vi "Check Formulas Alias Name.vi"(6 "Reserved Keywords":string[](array[string])=["All_Photons", "F_D^D", "F_D^_A", "F_A^_D", "F_A^A", "F_D^M", "F_A^M", "Donor", "Acceptor", "FRET", "ALEX", "t_burst", "B_All", "B_D^D", "B_D^A", "B_A^D", "B_A^A", "B^D", "B^A"], 8 "Descriptions Array in":string[](array[string]), 9 "Definitions Array in":string[](array[string]), 10 "Aliases Array in":string[](array[string]), 11 "Alias Definition":T1) -> (0 "Descriptions Array out":string[](array[string]), 1 "Definitions Array out":string[](array[string]), 2 "Aliases Array out":string[](array[string]), 3 "Selected Alias":i32)   [LabVIEW 2021, in "Formula.lvlib"]
uses:
  Formula.lvlib
  Formula Alias Definition.ctl
  GUI/GUI.lvlib
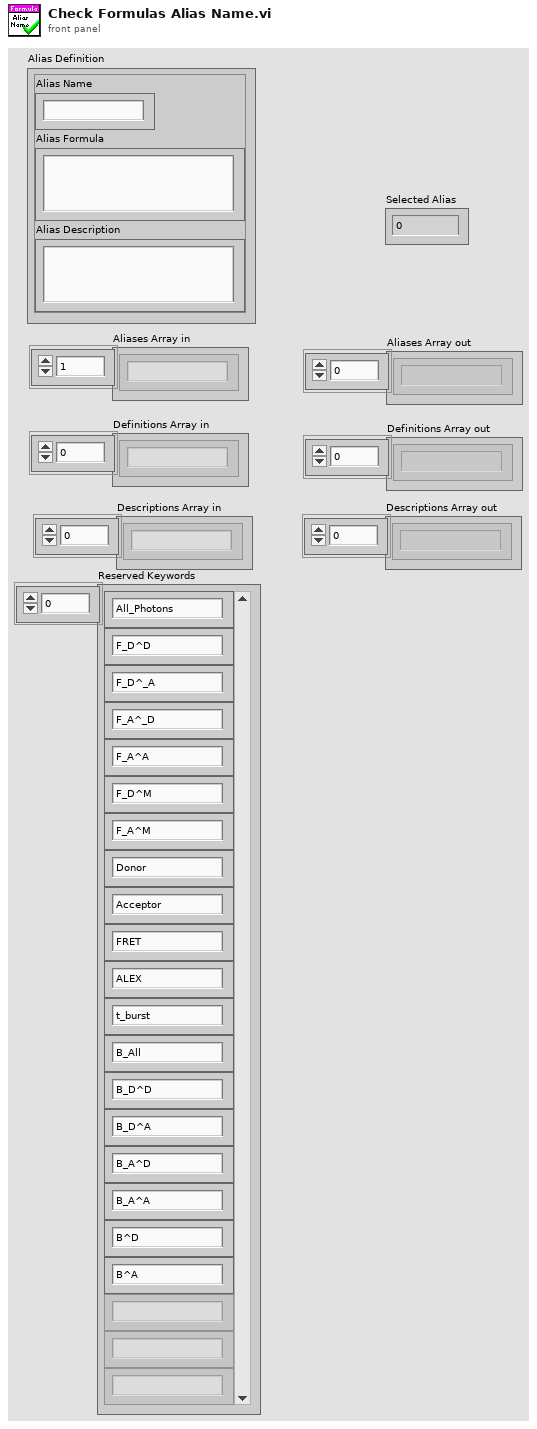
[diagram p1: front panel]
types:
  T1 = typedef "Formula.lvlib/Formula Alias Definition.ctl" = cluster{"Alias Formula":string, "Alias Name":string, "Alias Description":string}
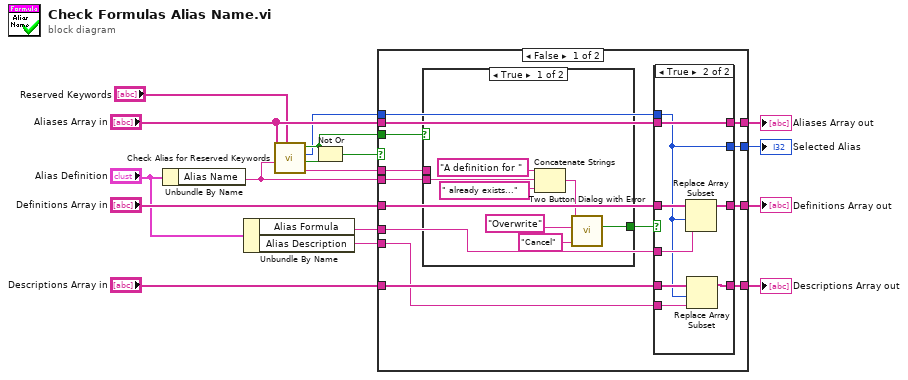
[diagram p0: block diagram]
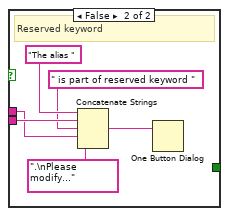
[diagram p2: hidden frame]
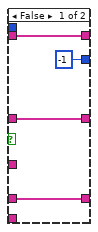
[diagram p3: hidden frame]
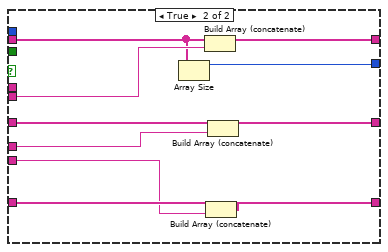
[diagram p4: hidden frame]
diagram:
  n1 = Unbundle By Name("Alias Definition") -> ("Alias Name"=w2:string)
  n2 = Unbundle By Name("Alias Definition") -> ("Alias Formula"=w6:string, "Alias Description"=w4:string)
  n3 = call "Check Alias for Reserved Keywords.vi"("Reserved Keywords"="Reserved Keywords", "Alias Name"=w2, "Aliases Array in"="Aliases Array in") -> ("Keyword"=w9:string, "Is Part of Reserved Keywords"=w11:bool, "index of element"=w8:i32, "Duplicate"=w10:bool)  [unwired: 5 in]
  n4 = Not Or(1:w11, 2:w10) -> (0:w12:bool)
  n5 = case shown="False" w12 {
    tunnel: "Aliases Array in" -> [w29 w61]
    tunnel: w2 -> [w31 w66]
    tunnel: "Definitions Array in" -> [w27 w65]
    tunnel: w6 -> [w25 w64]
    tunnel: [w28 w63] -> w15
    tunnel: [w26 w62] -> w14
    tunnel: [w24 w60] -> w13
    tunnel: w10 -> [w23 _]
    tunnel: w9 -> [w22 _]
    tunnel: w8 -> [w21 _]
    tunnel: "Descriptions Array in" -> [w20 w59]
    tunnel: w4 -> [w18 w58]
    tunnel: [w19 w57] -> w3
    frame False {
      n6 = case shown="True" w23 {
        tunnel: w31 -> [w38 w44]
        tunnel: [w34 _] -> w30
        tunnel: w22 -> [_ w39]
        frame True {
          n7 = Concatenate Strings("A definition for " ("string"), w38, " already exists..." ("string")) -> (w37:string)
          n8 = call "Two Button Dialog with Error.vi"("F button name (\"Cancel\")"="Cancel" ("F button name (\"Cancel\")"), "T button name (\"OK\")"="Overwrite" ("T button name (\"OK\")"), "message"=w37) -> ("T button?"=w34:bool)  [unwired: 7 in, 1 out]
        }
        frame False {
          # "Reserved keyword"
          n9 = Concatenate Strings("The alias " ("string"), w44, " is part of reserved keyword " ("string"), w39, ".\nPlease modify..." ("string")) -> (w41:string)
          n10 = One Button Dialog(message=w41) -> ()  [unwired: 1 in, 1 out]
        }
      }
      n11 = case shown="True" w30 {
        tunnel: w29 -> [w48 w56]
        tunnel: [w48 w56] -> w28
        tunnel: w27 -> [w47 w55]
        tunnel: [w47 w54] -> w26
        tunnel: w25 -> [_ w53]
        tunnel: [-1 ("index of element") w51] -> w24
        tunnel: w21 -> [_ w51]
        tunnel: w20 -> [w45 w52]
        tunnel: [w45 w50] -> w19
        tunnel: w18 -> [_ w49]
        frame False {
        }
        frame True {
          n12 = Replace Array Subset(array=w55, new element=w53, index=w51) -> (w54:string[])
          n13 = Replace Array Subset(array=w52, new element=w49, index=w51) -> (w50:string[])
        }
      }
    }
    frame True {
      n14 = Array Size(array=w61) -> (size(s)=w60:i32)
      n15 = Build Array (concatenate)(w61, w66) -> (w63:string[])
      n16 = Build Array (concatenate)(w59, w58) -> (w57:string[])
      n17 = Build Array (concatenate)(w65, w64) -> (w62:string[])
    }
  }
  "Definitions Array out" <- w14
  "Aliases Array out" <- w15
  "Selected Alias" <- w13
  "Descriptions Array out" <- w3
